vi "Convert_AC_FreqPct.vi"(1 "Freq_Hz":dbl[unit]) -> (0 "Freq%":dbl)   [LabVIEW 2024]
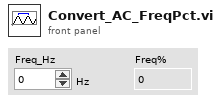
[diagram p1: front panel]
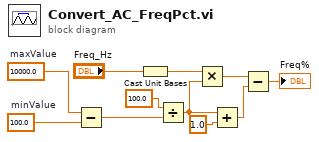
[diagram p0: block diagram]
diagram:
  w10 = 10000.0  # maxValue
  w5 = 100.0  # minValue
  n1 = Subtract(x=w10, y=w5) -> (x-y=w9:dbl)
  n2 = Cast Unit Bases(0:"Freq_Hz") -> (2:w6:dbl)  [unwired: 1 in]
  n3 = Divide(x=100.0, y=w9) -> (x/y=w3:dbl)
  n4 = Multiply(x=w6, y=w3) -> (x*y=w11:dbl)
  n5 = Add(x=w3, y=1.0) -> (x+y=w2:dbl)
  n6 = Subtract(x=w11, y=w2) -> (x-y=→"Freq%":dbl)
